vi "Query Event Log Selected Entries.vi"(8 "error in (no error)":errorcluster, 9 "End Timestamp (\"2011,3,20,14,5,30,999\")":string="2011,3,20,14,5,30,999", 10 "Start Timestamp (\"2011,3,20,12,5,30,999\")":string="2011,3,20,12,5,30,999", 11 "VISA resource name":refnum<visa-resource-name>) -> (0 "error out":errorcluster, 3 "VISA resource name out":refnum<visa-resource-name>)   [LabVIEW 2015, in "Rohde&Schwarz CMXP Base.lvlib"]
doc: "Queries all event log entries with a timestamp between the Start timestamp and End timestamp.\n\nFor each relevant entry, three parameters are returned: {<Severity>, <Timestamp>, <Message>}entry 1, {<Severity>, <Timestamp>, <Message>}entry 2, ...\n\nAttribute:\n-\n\nRemote-control command:\nSENSe:ELOG:TIME?"
uses:
  <instrlib>/Rohde&Schwarz CMXP Base/Rohde&Schwarz CMXP Base.lvlib
  <instrlib>/Rohde&Schwarz CMXP Base/Private/rsidr_core.llb/rsidr_core.lvlib
panel:
  out "Event Logs":T1(array[cluster])
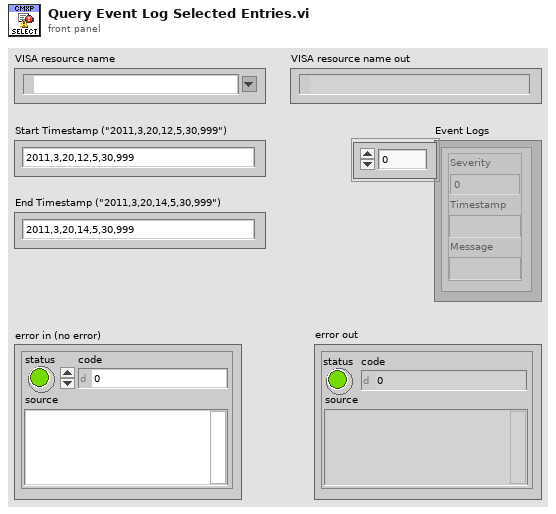
[diagram p1: front panel]
types:
  T1 = cluster{"Severity":dbl, "Timestamp":string, "Message":string}[]
  T2 = cluster{"Severity":i32, "Timestamp":string, "Message":string}
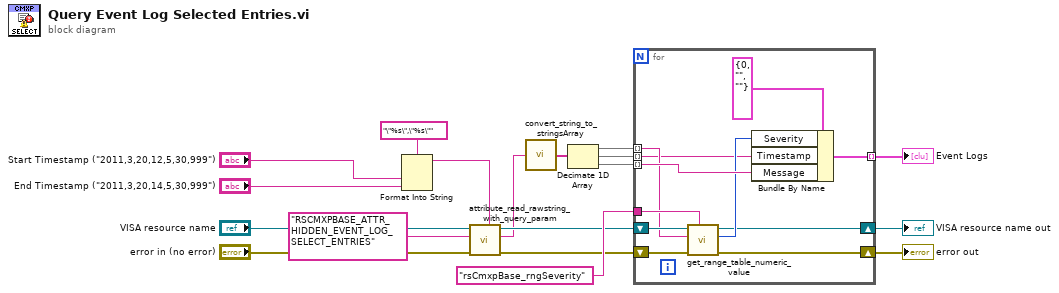
[diagram p0: block diagram]
diagram:
  n1 = Format Into String(format string="\"%s\",\"%s\"", "Start Timestamp (\"2011,3,20,12,5,30,999\")", "End Timestamp (\"2011,3,20,14,5,30,999\")") -> (resulting string=w5:string)  [unwired: 2 in, 1 out]
  n2 = call <instrlib>:"attribute_read_rawstring_with_query_param.vi"("Query Parameter (None)"=w5, "error in"="error in (no error)", "Attribute ID"="RSCMXPBASE_ATTR_HIDDEN_EVENT_LOG_SELECT_ENTRIES", "VISA resource name"="VISA resource name") -> ("error out"=w9:errorcluster, "RawString out"=w4:string, "VISA resource name out"=w10:refnum<visa-resource-name>)  [unwired: 5 in]
  n3 = call <instrlib>:"convert_string_to_stringsArray.vi"("String in"=w4) -> ("string array out"=w18:string[])  [unwired: 3 in, 1 out]
  n4 = Decimate 1D Array(w18) -> (w17:string[], w16:string[], w11:string[])
  n5 = for {
    tunnel: w17 -> [w23] mode=indexing
    tunnel: w16 -> [w19] mode=indexing
    tunnel: w11 -> [w28] mode=indexing
    tunnel: [w27] -> w12 mode=indexing
    tunnel: "rsCmxpBase_rngSeverity" ("Range Table ID in") -> [w24]
    shift-right: [w20] -> w14
    shift-left: w10 -> [w25]
    shift-right: [w21] -> w13
    shift-left: w9 -> [w26]
    n6 = call <instrlib>:"get_range_table_numeric_value.vi"("Range Table ID in"=w24, "error in"=w26, "String Value"=w23, "VISA resource name"=w25) -> ("error out"=w21:errorcluster, "I32 output"=w22:i32, "VISA resource name out"=w20:refnum<visa-resource-name>)  [unwired: 5 in]
    n7 = Bundle By Name(cluster=T2 {"Severity"=0, "Timestamp"="", "Message"=""} ("Event Logs 2"), "Severity"=w22, "Timestamp"=w19, "Message"=w28) -> (w27:T2)
  }
  "error out" <- w13
  "VISA resource name out" <- w14
  "Event Logs" <- w12
